vi "Buffer Initialize.vi"(8 "error in (no error)":errorcluster, 9 "Number Of Elements":i32[](array[numeric]), 10 "Sector Number":i32, 11 "1D U16 Group With ID DVR Queue in":refnum<class "2D U16 Group With ID DVR Queue.lvclass">) -> (0 "error out":errorcluster, 3 "1D U16 Group With ID DVR Queue out":refnum<class "2D U16 Group With ID DVR Queue.lvclass">)   [LabVIEW 2024, in "2D U16 Group With ID DVR Queue.lvclass"]
uses:
  2D U16 Group With ID DVR Queue.lvclass
  Type Def/Data Type.ctl
  2D U16 Group With ID DVR Queue.lvclass/2D U16 Group With ID DVR Queue.ctl
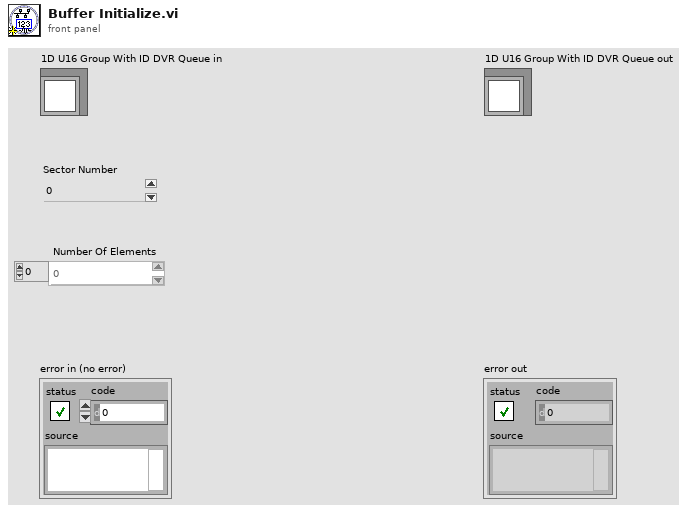
[diagram p1: front panel]
types:
  T1 = typedef "Data Type.ctl" = cluster{"Data ID":i64, "U16 Data Group":cluster{"Array":u16[][]}[]}
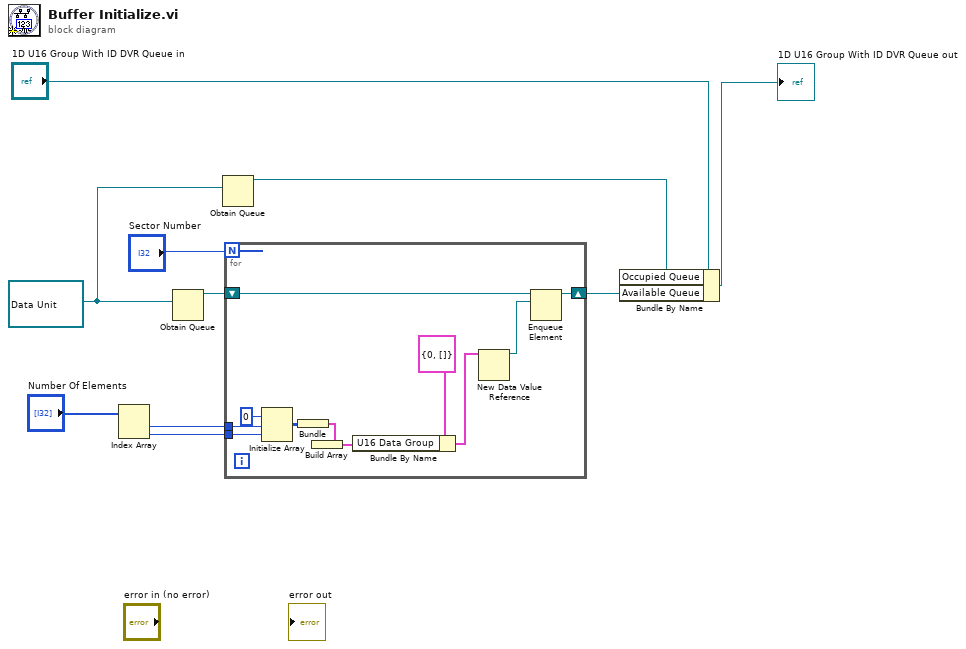
[diagram p0: block diagram]
diagram:
  w7 = refnum<data-value> refnum ("data value reference")
  n1 = Index Array(array="Number Of Elements") -> (element #1=w2:i32, element #2=w1:i32)  [unwired: 2 in]
  n2 = Obtain Queue(element data type=w7) -> (queue out=w10:refnum<queue>)  [unwired: 4 in, 2 out]
  n3 = Obtain Queue(element data type=w7) -> (queue out=w8:refnum<queue>)  [unwired: 4 in, 2 out]
  n4 = for {
    N: "Sector Number" -> [_]
    shift-right: [w20] -> w9
    shift-left: w10 -> [w21]
    tunnel: w2 -> [w19]
    tunnel: w1 -> [w18]
    n5 = Initialize Array(u16 0 ("element"), w19, w18) -> (w15:u16[][])
    n6 = Bundle(w15) -> (w14:cluster{u16[][]})  [unwired: 1 in]
    n7 = Build Array(w14) -> (w13:cluster{u16[][]}[])
    n8 = Bundle By Name(cluster=T1 {"Data ID"=0, "U16 Data Group"=[]} ("Data Unit"), "U16 Data Group"=w13) -> (w12:T1)
    n9 = New Data Value Reference(data value=w12) -> (data value reference=w11:refnum<data-value>)  [unwired: 1 in, 1 out]
    n10 = Enqueue Element(queue=w21, element=w11) -> (queue out=w20:refnum<queue>)  [unwired: 2 in, 2 out]
  }
  n11 = Bundle By Name(cluster="1D U16 Group With ID DVR Queue in", "Occupied Queue"=w8, "Available Queue"=w9) -> (→"1D U16 Group With ID DVR Queue out":refnum<class "2D U16 Group With ID DVR Queue.lvclass">)
